vi "Read Actor.vi"(11 "Base Actor in":refnum<class "Base Actor.lvclass">) -> (2 "Actor":refnum<class "Actor.lvclass">)   [LabVIEW 2025, in "jettl.lvlib" / "Base jettl Actor.lvlib" / "Base Actor.lvlib" / "Base Actor.lvclass"]
uses:
  Base Actor.lvclass
  Actor/Actor.lvclass
  Base Actor.lvclass/Base Actor.ctl
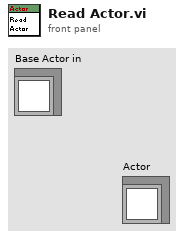
[diagram p1: front panel]
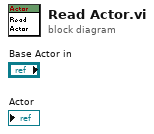
[diagram p0: block diagram]
diagram:
